vi "Simple Reader.vi"(8 "error in (no error)":errorcluster, 11 "Arduino Temperature Controller Driver in":refnum<class "Arduino Temperature Controller Driver.lvclass">) -> (0 "error out":errorcluster, 2 "Signals":dbl[](array[numeric]), 3 "Arduino Temperature Controller Driver out":refnum<class "Arduino Temperature Controller Driver.lvclass">)   [LabVIEW 2019, in "Arduino Temperature Controller Driver.lvclass"]
uses:
  Arduino Temperature Controller Driver.lvclass
  C:/GitHub/NHMFL_Core/Libraries/Instruments/VISA Instrument/VISA Instrument.lvclass
  C:/GitHub/NHMFL_Core/Libraries/Instruments/Temperature Controller Driver/Temperature Controller Driver.lvclass
  VISA Instrument/VISA Instrument.lvclass/VISA Instrument.ctl
  VISA Instrument/Read VISA resource.vi
  VISA Instrument/Write VISA resource.vi
  Temperature Controller Driver/Read T controller configuration.vi
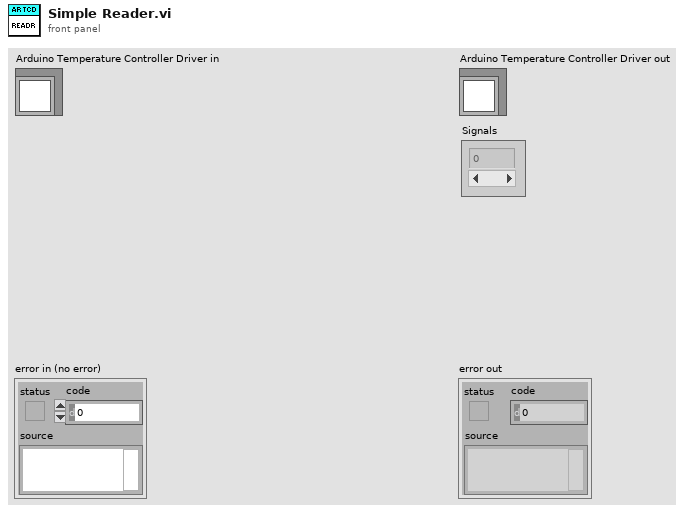
[diagram p1: front panel]
types:
  T1 = typedef "T controller configuration.ctl" = cluster{"Record Channels":string[], "Add raw signal":bool, "New set point":dbl, "Record heater":bool}
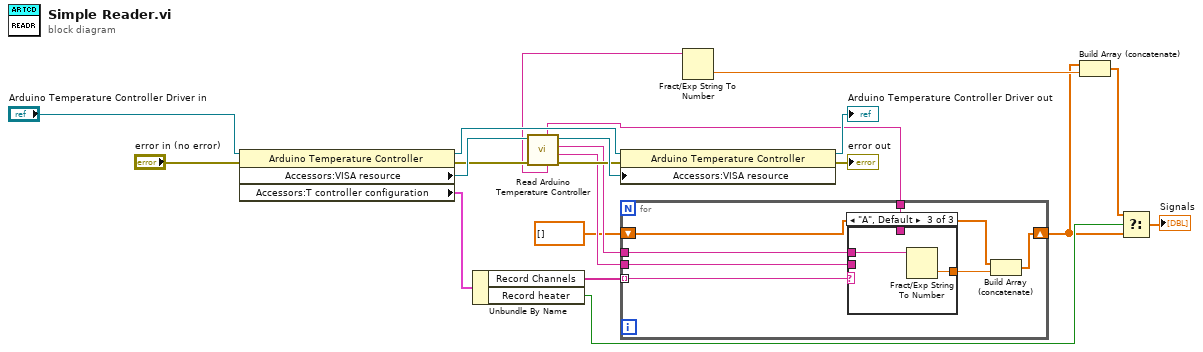
[diagram p0: block diagram]
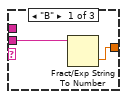
[diagram p2: hidden frame]
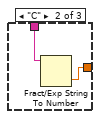
[diagram p3: hidden frame]
diagram:
  n1 = property class="Arduino Temperature Controller "(reference="Arduino Temperature Controller Driver in", error in="error in (no error)") -> (reference out=w19:refnum<class "Arduino Temperature Controller Driver.lvclass">, error out=w13:errorcluster, "Accessors:VISA resource"=w14:refnum<visa-resource-name>, "Accessors:T controller configuration"=w20:T1)
  n2 = Unbundle By Name(w20) -> ("Record Channels"=w21:string[], "Record heater"=w7:bool)
  n3 = call "Read Arduino Temperature Controller.vi"("Error In"=w13, "VISA resource name"=w14) -> ("Error Out"=w11:errorcluster, "Control temperature"=w9:string, "Sample temperature"=w10:string, "VISA resource name out"=w12:refnum<visa-resource-name>, "Power"=w6:string, "Set point"=w1:string)  [unwired: 4 in]
  n4 = property class="Arduino Temperature Controller "(reference=w19, error in=w11, "Accessors:VISA resource"=w12) -> (reference out=→"Arduino Temperature Controller Driver out":refnum<class "Arduino Temperature Controller Driver.lvclass">, error out=→"error out":errorcluster)
  n5 = for {
    tunnel: w21 -> [w28] mode=indexing
    tunnel: w10 -> [w27]
    shift-right: [w26] -> w3
    shift-left: dbl[] [] -> [w23]
    tunnel: w9 -> [w24]
    tunnel: w1 -> [w22]
    n6 = case shown="\"A\", Default" w28 {
      tunnel: w27 -> [_ _ w34]
      tunnel: [w29 w32 w33] -> w25
      tunnel: w24 -> [w30 _ _]
      tunnel: w22 -> [_ w31 _]
      frame "B" {
        n7 = Fract/Exp String To Number(string=w30) -> (number=w29:dbl)  [unwired: 3 in, 1 out]
      }
      frame "C" {
        n8 = Fract/Exp String To Number(string=w31) -> (number=w32:dbl)  [unwired: 3 in, 1 out]
      }
      frame "A", Default {
        n9 = Fract/Exp String To Number(string=w34) -> (number=w33:dbl)  [unwired: 3 in, 1 out]
      }
    }
    n10 = Build Array (concatenate)(w23, w25) -> (w26:dbl[])
  }
  n11 = Fract/Exp String To Number(string=w6) -> (number=w5:dbl)  [unwired: 3 in, 1 out]
  n12 = Build Array (concatenate)(w3, w5) -> (w4:dbl[])
  n13 = Select(t=w4, s=w7, f=w3) -> (s? t:f=→"Signals":dbl[])
